vi "Cálculos não uniforme.vi"(0 "Dados in":T2, 1 "Infos para processamento in":T1={"Diâmetro do furo [mm]"=1.4, "Diâmetro da linha média [mm]"=5.0, "IncF"=0.2, "Módulo de elasticidade [GPa]"=207.0, "Módulo de Poisson"=0.3, "Tipo de roseta utilizada"=enum."Tipo A", "Método de análise"=enum."Simplificado 2008", "Pfinal"=0.3, "Parar auto."=TRUE}) -> (2 "Círculo de Mohr":cluster{"Array":dbl[], "Array":dbl[]}[][](array[cluster]), 3 "Resultados":dbl[][](array[numeric]), 4 "Resultados médios":string[][](array[string]))   [LabVIEW 2016]
uses:
  Controles/p,q, t, a e b.ctl
  Controles/Infos para processamento.ctl
  <vilib>/Analysis/baseanly.llb/Mean (DBL).vi
  <vilib>/gmath/NI_Gmath.lvlib
  <vilib>/Analysis/NI_AALBase.lvlib
panel:
  out "Iterações":i32
  out "Coeficientes de controle":dbl[](array[numeric])
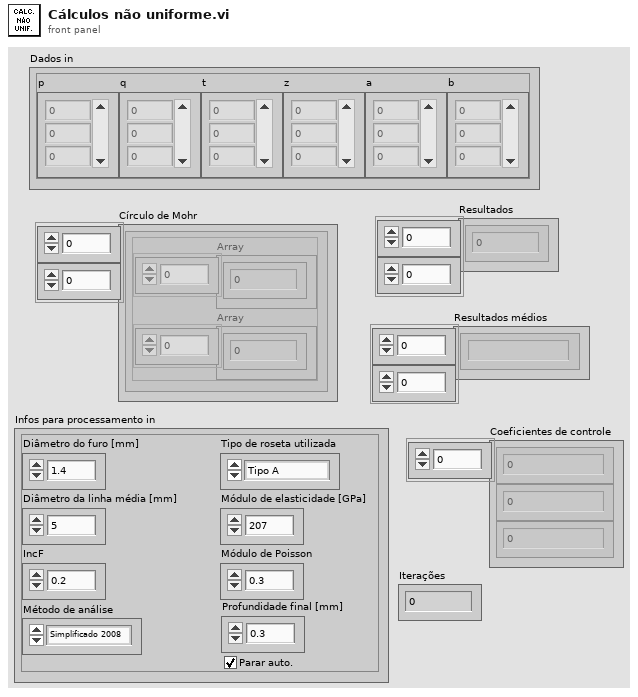
[diagram p1: front panel]
types:
  T1 = typedef "Infos para processamento.ctl" = cluster{"Diâmetro do furo [mm]":dbl, "Diâmetro da linha média [mm]":dbl, "IncF":dbl, "Módulo de elasticidade [GPa]":dbl, "Módulo de Poisson":dbl, "Tipo de roseta utilizada":enum16{"Tipo A", "Tipo B", "Tipo C"}, "Método de análise":enum16{"Não uniforme 2013", "Simplificado 2013", "Simplificado 2008"}, "Pfinal":dbl, "Parar auto.":bool}
  T2 = typedef "p,q, t, a e b.ctl" = cluster{"p":dbl[], "q":dbl[], "t":dbl[], "z":dbl[], "a":dbl[], "b":dbl[]}
  T3 = typedef "Matrizes não uniforme.ctl" = cluster{"aT":dbl[][], "bT":dbl[][], "aTa":dbl[][], "bTb":dbl[][]}
  T4 = typedef "Resultados não uniformes.ctl" = cluster{"P":dbl[], "Q":dbl[], "T":dbl[], "P rms":dbl, "Q rms":dbl, "T rms":dbl}
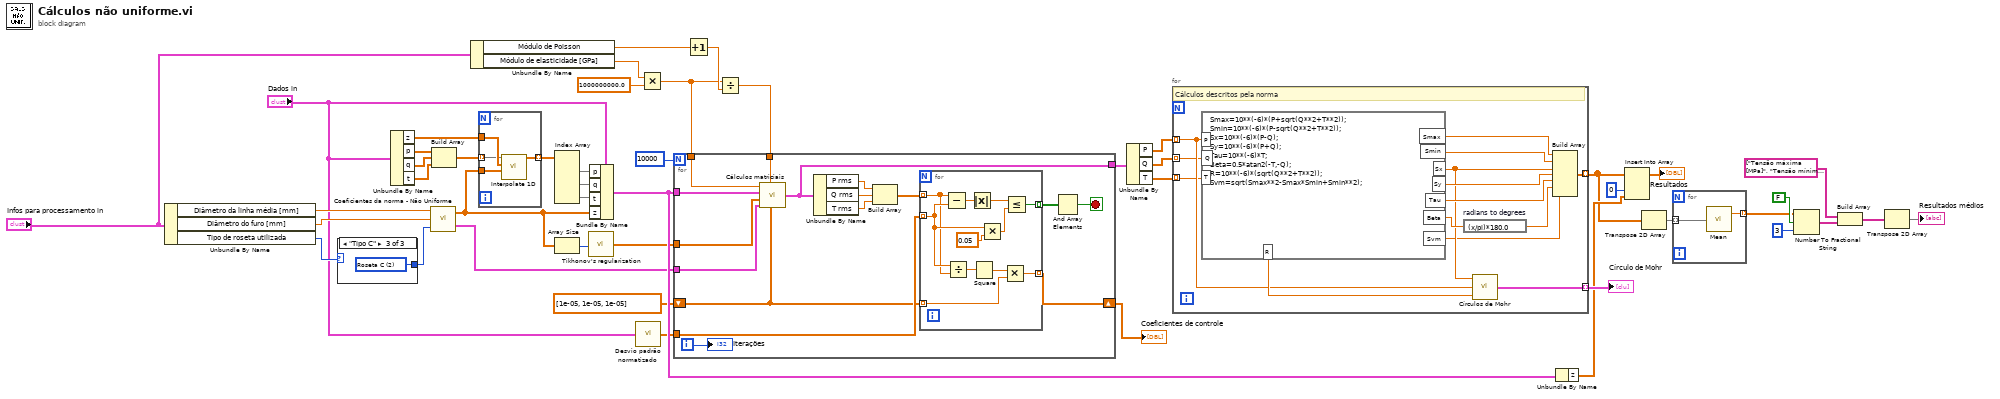
[diagram p0: block diagram]
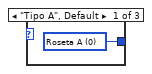
[diagram p2: hidden frame]
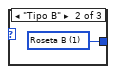
[diagram p3: hidden frame]
diagram:
  n1 = Unbundle By Name("Infos para processamento in") -> ("Diâmetro da linha média [mm]"=w22:dbl, "Diâmetro do furo [mm]"=w21:dbl, "Tipo de roseta utilizada"=w20:enum16{"Tipo A", "Tipo B", "Tipo C"})
  n2 = case shown="\"Tipo C\"" w20 {
    tunnel: [w48 w49 w50] -> w19
    frame "Tipo A", Default {
      w48 = u16 0 items=["Roseta A", "Roseta B", "Roseta C"] ("Tipo de roseta")
    }
    frame "Tipo B" {
      w49 = u16 1 items=["Roseta A", "Roseta B", "Roseta C"] ("Tipo de roseta")
    }
    frame "Tipo C" {
      w50 = u16 2 items=["Roseta A", "Roseta B", "Roseta C"] ("Tipo de roseta")
    }
  }
  n3 = Unbundle By Name("Dados in") -> ("z"=w46:dbl[], "p"=w45:dbl[], "q"=w44:dbl[], "t"=w43:dbl[])
  n4 = call "Coeficientes da norma - Não Uniforme.vi"("Tipo de roseta"=w19, "Diâmetro do furo"=w21, "Diâmetro da roseta"=w22) -> ("Matrizes"=w33:T3, "Vetor das medidas"=w5:dbl[])
  n5 = Build Array(w45, w44, w43) -> (w42:dbl[][])
  n6 = Unbundle By Name("Infos para processamento in") -> ("Módulo de Poisson"=w17:dbl, "Módulo de elasticidade [GPa]"=w16:dbl)
  n7 = for {
    tunnel: w46 -> [w54]
    tunnel: w5 -> [w53]
    tunnel: w42 -> [w52] mode=indexing
    tunnel: [w51] -> w41 mode=indexing
    n8 = call <vilib>:"Interpolate 1D.vi"("xi"=w53, "X"=w54, "Y"=w52) -> ("yi"=w51:dbl[])  [unwired: 6 in, 2 out]
  }
  n9 = Index Array(array=w41) -> (element #1=w40:dbl[], element #2=w39:dbl[], element #3=w38:dbl[])  [unwired: 6 in]
  n10 = Array Size(array=w5) -> (size(s)=w37:i32)
  n11 = call "Tikhonov's regularization.vi"("Ordem"=w37) -> ("Matriz de regularização"=w34:dbl[][])
  n12 = Bundle By Name(cluster="Dados in", "p"=w40, "q"=w39, "t"=w38, "z"=w5) -> (w47:T2)
  n13 = call "Desvio padrão normatizado.vi"("Dados out"="Dados in") -> ("Desvios das deformações"=w30:dbl[])
  n14 = Multiply(x=w16, y=1000000000.0) -> (x*y=w15:dbl)
  n15 = Increment(x=w17) -> (x+1=w35:dbl)
  n16 = Divide(x=w15, y=w35) -> (x/y=w32:dbl)
  n17 = for {
    N: 10000 -> [_]
    tunnel: w34 -> [w66]
    tunnel: w47 -> [w70]
    tunnel: w33 -> [w69]
    tunnel: w32 -> [w68]
    tunnel: w15 -> [w67]
    shift-right: [w57] -> w6
    shift-left: dbl[] [1e-05, 1e-05, 1e-05] ("Coeficientes de controle") -> [w58]
    tunnel: w30 -> [w61]
    tunnel: [w56] -> w26
    i -> [w55]
    stop <- w59 stop-if-true
    n18 = call "Cálculos matriciais.vi"("Coeficientes de controle"=w58, "G"=w68, "Matrizes"=w69, "Matriz de regularização"=w66, "Dados in"=w70, "E"=w67) -> ("Resultados"=w56:T4)
    n19 = Unbundle By Name(w56) -> ("P rms"=w65:dbl, "Q rms"=w64:dbl, "T rms"=w63:dbl)
    n20 = Build Array(w65, w64, w63) -> (w62:dbl[])
    n21 = for {
      tunnel: w62 -> [w77] mode=indexing
      tunnel: w61 -> [w78] mode=indexing
      tunnel: [w79] -> w60 mode=indexing
      tunnel: w58 -> [w74] mode=indexing
      tunnel: [w73] -> w57 mode=indexing
      n22 = Subtract(x=w77, y=w78) -> (x-y=w81:dbl)
      n23 = Divide(x=w78, y=w77) -> (x/y=w76:dbl)
      n24 = Absolute Value(x=w81) -> (abs(x)=w71:dbl)
      n25 = Square(x=w76) -> (x^2=w75:dbl)
      n26 = Multiply(x=w78, y=0.05) -> (x*y=w72:dbl)
      n27 = Multiply(x=w75, y=w74) -> (x*y=w73:dbl)
      n28 = Less Or Equal?(x=w71, y=w72) -> (x <= y?=w79:bool)
    }
    n29 = And Array Elements(Boolean array=w60) -> (logical AND=w59:bool)
    "Iterações" <- w55
  }
  "Coeficientes de controle" <- w6
  n30 = Unbundle By Name(w26) -> ("P"=w25:dbl[], "Q"=w24:dbl[], "T"=w23:dbl[])
  n31 = for {
    tunnel: w25 -> [w84] mode=indexing
    tunnel: w24 -> [w83] mode=indexing
    tunnel: w23 -> [w82] mode=indexing
    tunnel: [w93] -> w1 mode=indexing
    tunnel: [w86] -> w29 mode=indexing
    # "Cálculos descritos pela norma"
    n32 = formula code="Smax=10**(-6)*(P+sqrt(Q**2+T**2));\nSmin=10**(-6)*(P-sqrt(Q**2+T**2));\nSx=10**(-6)*(P-Q);\nSy=10**(-6)*(P+Q);\nTau=10**(-6)*T;\nBeta=0.5*atan2(-T,-Q);\nR=10**(-6)*(sqrt(Q**2+T**2));\nSvm=sqrt(Smax**2-Smax*Smin+Smin**2);"("P"=w84, "Q"=w83, "T"=w82) -> ("Smax"=w92:dbl, "Smin"=w91:dbl, "Sx"=w88:dbl, "Sy"=w95:dbl, "Tau"=w94:dbl, "Beta"=w90:dbl, "R"=w87:dbl, "Svm"=w85:dbl)
    n33 = expression code="(x/pi)*180.0" "radians to degrees"(w90) -> (w89:dbl)
    n34 = call "Círculos de Mohr.vi"("R"=w87, "P"=w84, "Sx"=w88) -> ("Círculo de Mohr"=w86:cluster{"Array":dbl[], "Array":dbl[]}[])
    n35 = Build Array(w92, w91, w88, w95, w94, w89, w85) -> (w93:dbl[])
  }
  "Círculo de Mohr" <- w29
  n36 = Unbundle By Name(w47) -> ("z"=w2:dbl[])
  n37 = Insert Into Array(array=w1, index (col)=0 ("disabled index (col)"), new element=w2) -> (→"Resultados":dbl[][])  [unwired: 1 in]
  n38 = Transpose 2D Array(2D array=w1) -> (transposed array=w3:dbl[][])
  n39 = for {
    tunnel: w3 -> [w96] mode=indexing
    tunnel: [w97] -> w7 mode=indexing
    n40 = call-poly <vilib>:"Mean.vi"("X"=w96) -> ("mean"=w97:dbl)  [unwired: 1 out]
  }
  n41 = Number To Fractional String(use system decimal point (T)=FALSE, number=w7, precision (6)=i16 3) -> (F-format string=w11:string[])  [unwired: 1 in]
  n42 = Build Array(string[] ["Tensão máxima [MPa]", "Tensão mínima [MPa]", "Tensão em x [MPa]", "Tensão em y [MPa]", "Tensão cisalhante [MPa]", "Ângulo da tensão máxima [°]", "Tensão de von Misses [MPa]"] ("element"), w11) -> (w9:string[][])
  n43 = Transpose 2D Array(2D array=w9) -> (transposed array=→"Resultados médios":string[][])
